vi "E8267D SetFrequency.vi"(0 "VISA Rsrc":refnum<visa-resource-name>="GPIB0::12::INSTR", 5 "Frequency (Hz)":dbl, 7 "FUnits":u16(ring) caption="Units" items=["Hz", "MHz", "GHz"], 11 "error in (no error)":errorcluster) -> (4 "VISA Rsrc Out":refnum<visa-resource-name>="GPIB0::12::INSTR", 15 "error out":errorcluster)   [LabVIEW 2019]
doc: "Ce VI écrit les paramètres de la zone de contrôle spécifiée dans le contrôlleur"
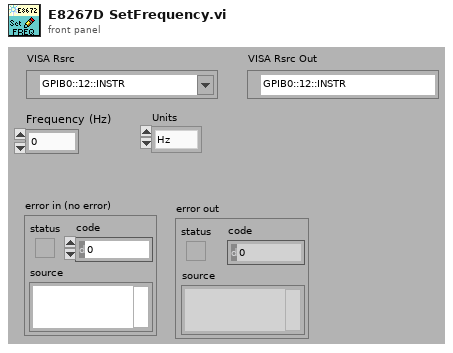
[diagram p1: front panel]
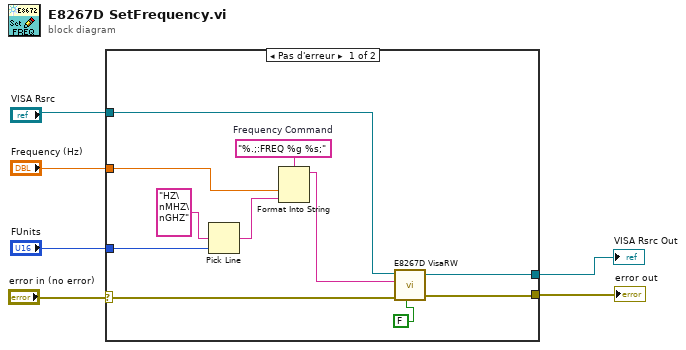
[diagram p0: block diagram]
diagram:
  n1 = case shown="Pas d'erreur" "error in (no error)" {
    selector: "error in (no error)" -> [w16 w19]
    tunnel: "VISA Rsrc" -> [w15 w18]
    tunnel: [w17 w19] -> w5
    tunnel: "Frequency (Hz)" -> [w9 _]
    tunnel: [w13 w18] -> w2
    tunnel: "FUnits" -> [w8 _]
    frame No Error {
      w12 = "%.;:FREQ %g %s;"  # Frequency Command
      n2 = Pick Line(multi-line string="HZ\nMHZ\nGHZ", line index=w8) -> (output string=w11:string)  [unwired: 1 in]
      n3 = Format Into String(format string=w12, w9, w11) -> (resulting string=w7:string)  [unwired: 2 in, 1 out]
      n4 = call <userlib>:"E8267D VisaRW.vi"("Lecture?(T)"=FALSE, "error in (no error)"=w16, "ChaineCom"=w7, "VISA Rsrc"=w15) -> ("error out"=w17:errorcluster, "VISA Rsrc Out"=w13:refnum<visa-resource-name>)  [unwired: 3 in, 2 out]
    }
    frame Error {
    }
  }
  "error out" <- w5
  "VISA Rsrc Out" <- w2
